vi "Levelmeter_automatic_refill.vi"(0 "n_shield":i32=50 max=100 step=10, 1 "min_n_shield":i32=50 min=0 max=100 step=10, 2 "max_n_shield":i32=100 min=0 max=100 step=10, 3 "max filltime n_shield [min]":dbl=25.0, 4 "wait for n_shield [min]":dbl, 5 "LN Jacket Refill":bool, 6 "Automatic refill Jacket":bool, 7 "Automatic refill Coldtraps":bool=TRUE, 14 "n_cool":i32=50 max=100 step=10, 15 "min_n_cool":i32=50 min=0 max=100 step=10, 16 "max_n_cool":i32=100 min=0 max=100 step=10, 17 "max filltime n_cool [min]":dbl=10.0, 18 "wait for n_cool [min]":dbl=300.0, 19 "Coldtraps refill":bool) -> (8 "cool control":bool, 9 "shield control":bool, 10 "Übergabe LN Jacket refill":bool, 11 "Übergabe Coldtraps refill":bool)   [LabVIEW 2018]
uses:
  Global/Global Variables/Data_Display_global.vi
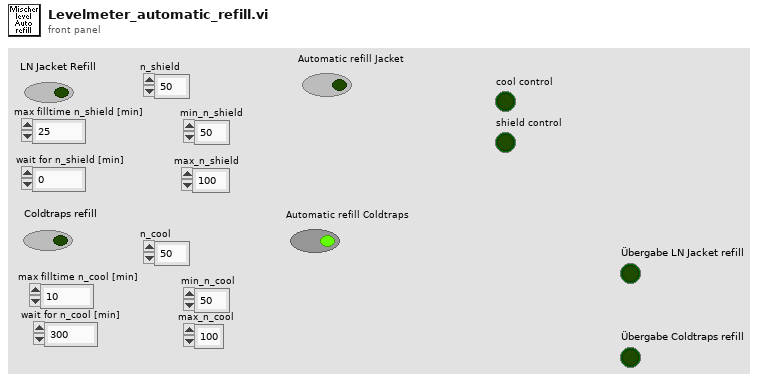
[diagram p1: front panel]
types:
  T1 = typedef "Mischer_Levelmeter-Cluster.ctl" = cluster{"Plot":dbl[][], "N-Shield (%)":dbl, "He (%)":dbl, "Coldtrap (%)":dbl, "He - POT (%)":dbl, "N-Shield Refill":bool, "Last fill Shield":string, "Auto Refill Shield":bool, "Trap Refill":bool, "Last fill Coldtrap":string, "Auto Refill Trap":bool, "Shield Refill":bool, "Coldtrap Refill":bool}
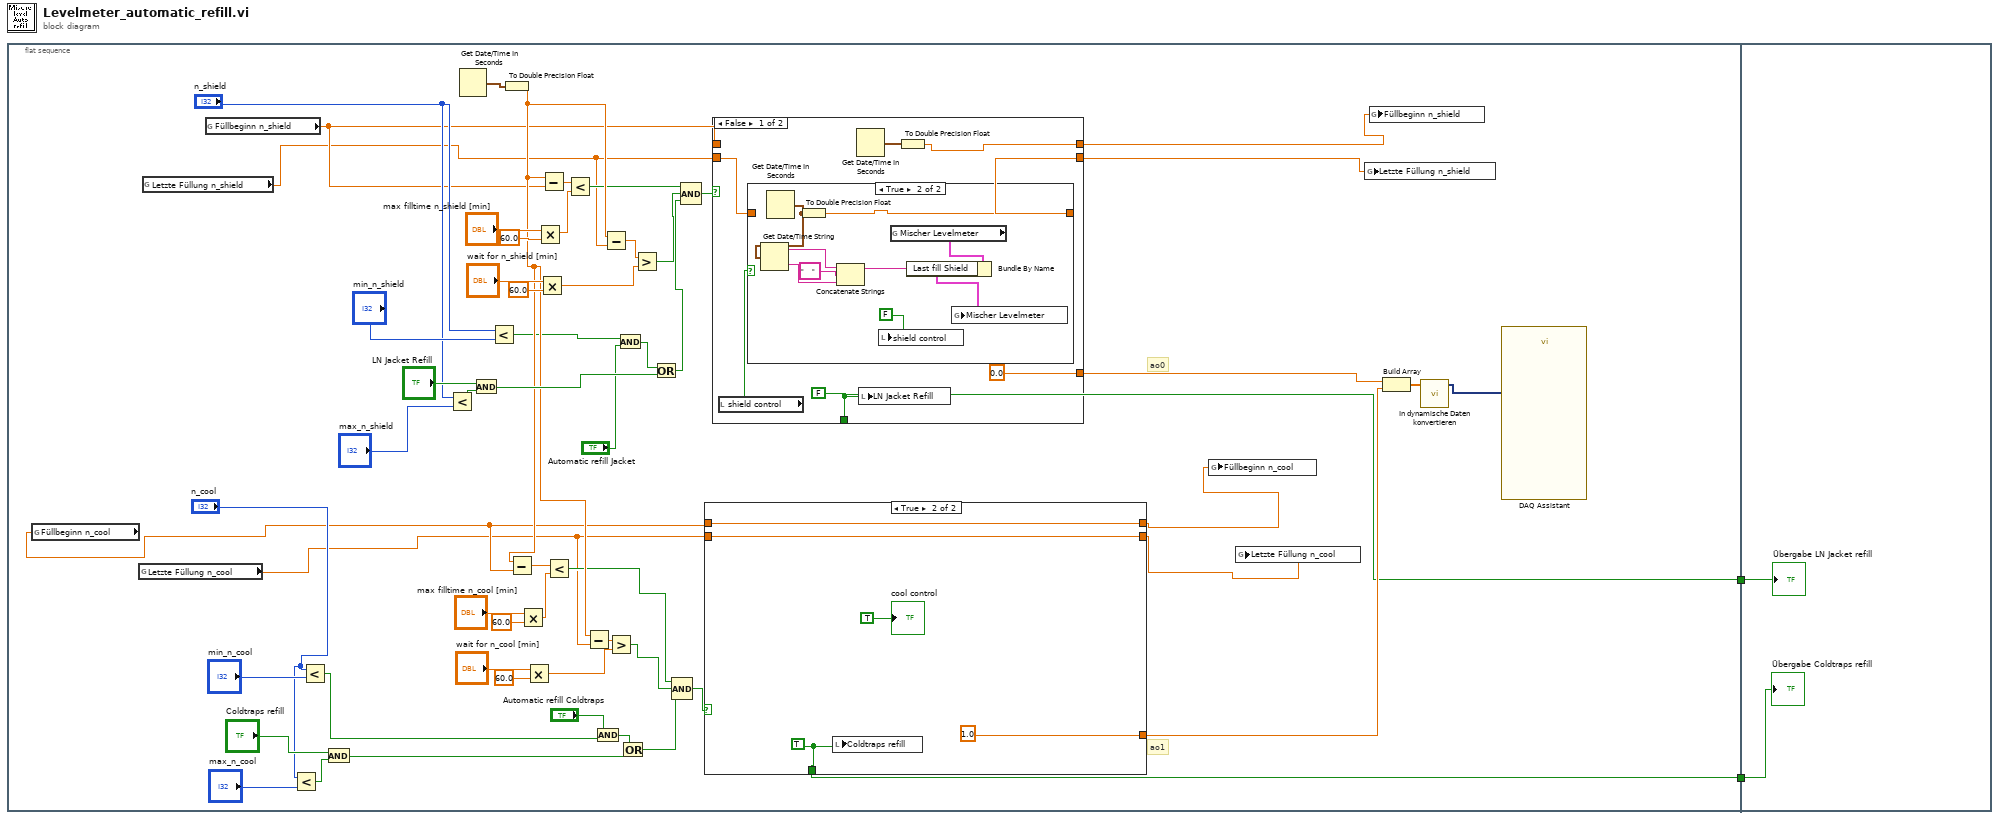
[diagram p0: block diagram]
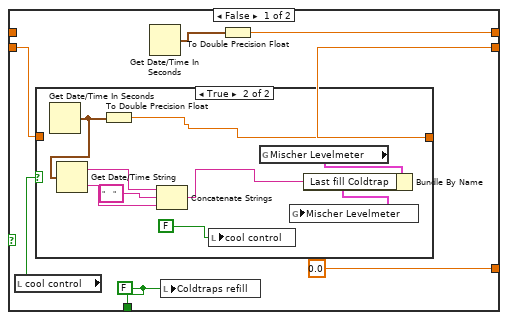
[diagram p2: hidden frame]
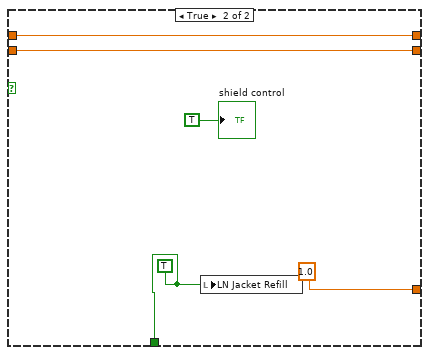
[diagram p5: hidden frame]
diagram:
  n1 = flat-sequence {
    tunnel: [w14] -> w2
    tunnel: [w13] -> w1
    tunnel: w2 -> [w106]
    tunnel: w1 -> [w105]
    frame #0 {
      # "ao1"
      # "ao0"
      n2 = global read "Data_Display_global.vi" "Füllbeginn n_cool"() -> (w5:dbl)
      n3 = global read "Data_Display_global.vi" "Letzte Füllung n_cool"() -> (w4:dbl)
      n4 = global read "Data_Display_global.vi" "Letzte Füllung n_shield"() -> (w9:dbl)
      n5 = global read "Data_Display_global.vi" "Füllbeginn n_shield"() -> (w10:dbl)
      n6 = Less?(x="n_cool", y="max_n_cool") -> (x < y?=w58:bool)
      n7 = Less?(x="n_cool", y="min_n_cool") -> (x < y?=w26:bool)
      n8 = And(x="Coldtraps refill", y=w58) -> (x .and. y?=w57:bool)
      n9 = Less?(x="n_shield", y="max_n_shield") -> (x < y?=w56:bool)
      n10 = Get Date/Time In Seconds() -> (seconds since 1Jan1904=w50:timestamp)
      n11 = And(x="LN Jacket Refill", y=w56) -> (x .and. y?=w51:bool)
      n12 = Less?(x="n_shield", y="min_n_shield") -> (x < y?=w30:bool)
      n13 = To Double Precision Float(number=w50) -> (double precision float=w35:dbl)
      n14 = Subtract(x=w35, y=w5) -> (x-y=w39:dbl)
      n15 = Multiply(x="max filltime n_cool [min]", y=60.0) -> (x*y=w38:dbl)
      n16 = Multiply(x="wait for n_cool [min]", y=60.0) -> (x*y=w33:dbl)
      n17 = Multiply(x="max filltime n_shield [min]", y=60.0) -> (x*y=w46:dbl)
      n18 = Multiply(x="wait for n_shield [min]", y=60.0) -> (x*y=w44:dbl)
      n19 = Subtract(x=w35, y=w10) -> (x-y=w49:dbl)
      n20 = Less?(x=w39, y=w38) -> (x < y?=w16:bool)
      n21 = Less?(x=w49, y=w46) -> (x < y?=w18:bool)
      n22 = Subtract(x=w35, y=w4) -> (x-y=w34:dbl)
      n23 = And(x="Automatic refill Coldtraps", y=w26) -> (x .and. y?=w27:bool)
      n24 = Subtract(x=w35, y=w9) -> (x-y=w45:dbl)
      n25 = Greater?(x=w34, y=w33) -> (0:w15:bool)
      n26 = And(x=w30, y="Automatic refill Jacket") -> (x .and. y?=w29:bool)
      n27 = Or(x=w27, y=w57) -> (x .or. y?=w41:bool)
      n28 = Greater?(x=w45, y=w44) -> (0:w17:bool)
      n29 = Or(x=w29, y=w51) -> (x .or. y?=w19:bool)
      n30 = Compound Arithmetic op=AND(w16, w15, w41) -> (w40:bool)
      n31 = Compound Arithmetic op=AND(w18, w17, w19) -> (w20:bool)
      n32 = case shown="True" w40 {
        tunnel: [0.0 ("Daten") 1.0 ("Daten")] -> w24
        tunnel: [w65 w80] -> w6
        tunnel: [w62 w81] -> w7
        tunnel: w5 -> [_ w81]
        tunnel: w4 -> [w66 w80]
        tunnel: [w61 w79] -> w14
        frame False {
          w61 = FALSE
          n33 = local read "cool control"() -> (w64:bool)
          n34 = case shown="True" w64 {
            tunnel: [w68 w73] -> w65
            tunnel: w66 -> [w68 _]
            frame False {
            }
            frame True {
              n35 = Get Date/Time In Seconds() -> (seconds since 1Jan1904=w74:timestamp)
              n36 = Get Date/Time String(seconds (now)=w74) -> (date string=w75:string, time string=w76:string)  [unwired: 2 in]
              n37 = To Double Precision Float(number=w74) -> (double precision float=w73:dbl)
              n38 = Concatenate Strings(w75, "    ", w76) -> (w70:string)
              n39 = local write "cool control"(FALSE ("shield control")) -> ()
              n40 = global read "Data_Display_global.vi" "Mischer Levelmeter"() -> (w72:T1)
              n41 = Bundle By Name(cluster=w72, "Last fill Coldtrap"=w70) -> (w71:T1)
              n42 = global write "Data_Display_global.vi" "Mischer Levelmeter"(w71) -> ()
            }
          }
          n43 = Get Date/Time In Seconds() -> (seconds since 1Jan1904=w63:timestamp)
          n44 = local write "Coldtraps refill"(w61) -> ()
          n45 = To Double Precision Float(number=w63) -> (double precision float=w62:dbl)
        }
        frame True {
          w79 = TRUE
          n46 = local write "Coldtraps refill"(w79) -> ()
          "cool control" <- TRUE ("Boolean")
        }
      }
      n47 = case "Case-Struktur" shown="False" w20 {
        tunnel: [0.0 ("Daten") 1.0 ("Daten")] -> w23
        tunnel: [w84 w103] -> w3
        tunnel: w10 -> [_ w103]
        tunnel: [w86 w101] -> w8
        tunnel: w9 -> [w85 w101]
        tunnel: [w83 w100] -> w13
        frame False {
          w83 = FALSE
          n48 = local read "shield control"() -> (w87:bool)
          n49 = case shown="True" w87 {
            tunnel: [w90 w95] -> w86
            tunnel: w85 -> [w90 _]
            frame False {
            }
            frame True {
              n50 = Get Date/Time In Seconds() -> (seconds since 1Jan1904=w96:timestamp)
              n51 = Get Date/Time String(seconds (now)=w96) -> (date string=w97:string, time string=w98:string)  [unwired: 2 in]
              n52 = To Double Precision Float(number=w96) -> (double precision float=w95:dbl)
              n53 = Concatenate Strings(w97, "    ", w98) -> (w92:string)
              n54 = local write "shield control"(FALSE ("shield control")) -> ()
              n55 = global read "Data_Display_global.vi" "Mischer Levelmeter"() -> (w94:T1)
              n56 = Bundle By Name(cluster=w94, "Last fill Shield"=w92) -> (w93:T1)
              n57 = global write "Data_Display_global.vi" "Mischer Levelmeter"(w93) -> ()
            }
          }
          n58 = Get Date/Time In Seconds() -> (seconds since 1Jan1904=w88:timestamp)
          n59 = local write "LN Jacket Refill"(w83) -> ()
          n60 = To Double Precision Float(number=w88) -> (double precision float=w84:dbl)
        }
        frame True {
          w100 = TRUE
          n61 = local write "LN Jacket Refill"(w100) -> ()
          "shield control" <- TRUE ("Boolean")
        }
      }
      n62 = global write "Data_Display_global.vi" "Füllbeginn n_cool"(w7) -> ()
      n63 = global write "Data_Display_global.vi" "Letzte Füllung n_cool"(w6) -> ()
      n64 = global write "Data_Display_global.vi" "Letzte Füllung n_shield"(w8) -> ()
      n65 = global write "Data_Display_global.vi" "Füllbeginn n_shield"(w3) -> ()
      n66 = Build Array(w23, w24) -> (w22:dbl[])
      n67 = call "In dynamische Daten konvertieren"("Array"=w22) -> ("Dynamic Data Type"=w21:dynamicdata)  [unwired: 3 in]
      n68 = call "DAQ Assistant"("data"=w21) -> ()  [unwired: 17 in, 2 out]
    }
    frame #1 {
      "Übergabe LN Jacket refill" <- w105
      "Übergabe Coldtraps refill" <- w106
    }
  }
